vi "read_4chFake.vi"(8 "previous value ch1":bool, 9 "pixel counter":u16, 11 "previous value ch0":bool) -> (0 "Inputl1":bool, 2 "read output":T1, 3 "Input0":bool)   [LabVIEW 2010]
uses:
  common_typedefs/channels_cluster.ctl
  <vilib>/eio/EIONode/EIONode.xnode
  <vilib>/rvi/eio/nirviEIOImplementation/nirviEIOImplementation.xnode
  <vilib>/rvi/eio/common/nirviEmuClasses.ctl
  <vilib>/rvi/eio/common/nirviEmuTemplateMethod_noerrors.vi
panel:
  out "Connector1/DIO1":bool
  out "Connector1/DIO23":bool
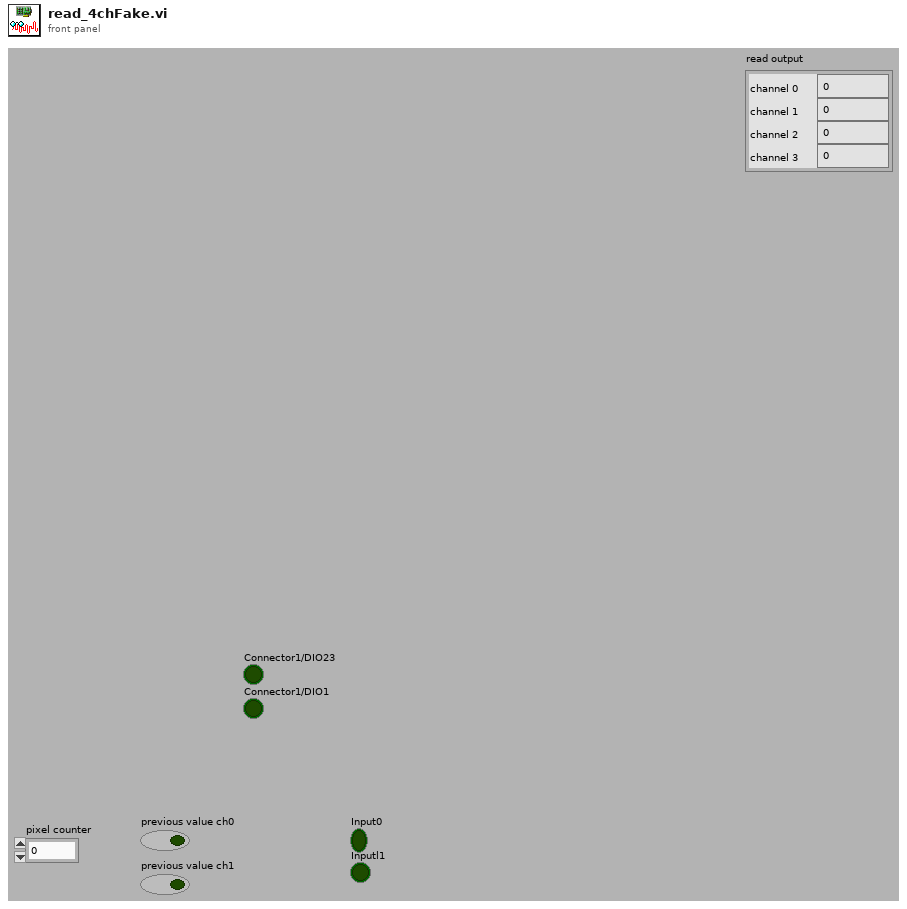
[diagram p1: front panel]
types:
  T1 = typedef "channels_cluster.ctl" = cluster{"channel 0":u32, "channel 1":u32, "channel 2":u32, "channel 3":u32}
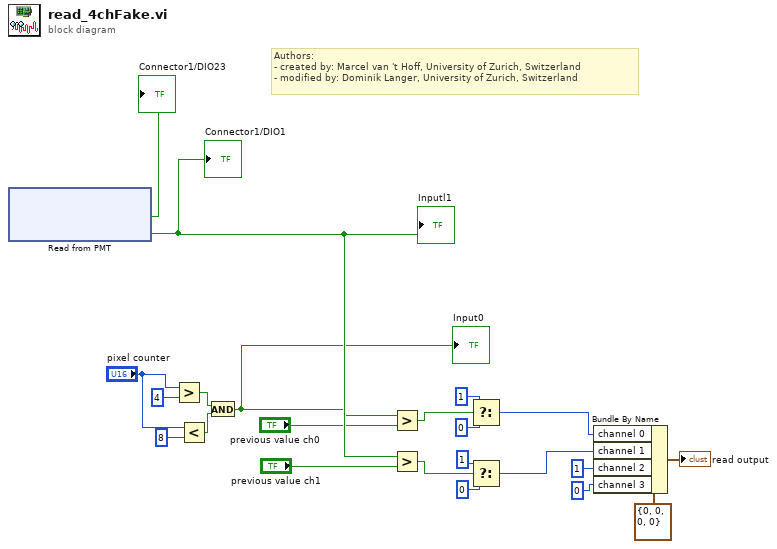
[diagram p0: block diagram]
diagram:
  # "Authors: \n- created by: Marcel van 't Hoff, University of Zurich, Switzerland\n- modified by: Dominik Langer, University of Zurich, Switzerland"
  n1 = xnode "Read from PMT"() -> ("Connector1/DIO23"=→"Connector1/DIO23":bool, "Connector1/DIO1"=w19:bool)  [unwired: 2 in, 2 out]
  "Inputl1" <- w19
  "Connector1/DIO1" <- w19
  n2 = Greater?(x="pixel counter", y=u16 4) -> (0:w3:bool)
  n3 = Less?(x="pixel counter", y=u16 8) -> (x < y?=w2:bool)
  n4 = And(x=w3, y=w2) -> (x .and. y?=w1:bool)
  "Input0" <- w1
  n5 = Greater?(x=w1, y="previous value ch0") -> (0:w12:bool)
  n6 = Greater?(x=w19, y="previous value ch1") -> (0:w11:bool)
  n7 = Select(t=u32 1, s=w12, f=u32 0) -> (s? t:f=w8:u32)
  n8 = Select(t=u32 1, s=w11, f=u32 0) -> (s? t:f=w7:u32)
  n9 = Bundle By Name(cluster=T1 {"channel 0"=0, "channel 1"=0, "channel 2"=0, "channel 3"=0} ("channel offsets 3"), "channel 0"=w8, "channel 1"=w7, "channel 2"=u32 1, "channel 3"=u32 0) -> (→"read output":T1)
